vi "Launcher.vi"   [LabVIEW 2015]
doc: "<b> </b> <b> </b>\n©2016 Q Software Innovations, LLC (QSI)\nwritten by Quentin Alldredge\nproduced in LabVIEW 2015"
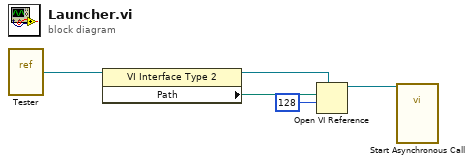
[diagram p0: block diagram]
diagram:
  n1 = vi-ref "Tester.vi"() -> (w5:refnum<vi>)
  n2 = property class="VI Interface Type 2"(reference=w5) -> (reference out=w3:refnum<vi>, "Path"=w4:path)  [unwired: 1 in, 1 out]
  n3 = Open VI Reference(type specifier VI Refnum (for type only)=w3, vi path=w4, options=128) -> (vi reference=w2:refnum<vi>)  [unwired: 3 in, 1 out]
  n4 = call-by-ref "Start Asynchronous Call"(reference=w2) -> ()  [unwired: 13 in, 2 out]
